vi "Forward SubVi.vi"(10 "Numeric":i32, 11 "Array":cluster{"Horizontal":i32, i32}[](array[cluster])) -> (2 "Cluster 2":cluster{"Horizontal":dbl, dbl}, 3 "Cluster":cluster{"Horizontal":i32, i32})   [LabVIEW 2014]
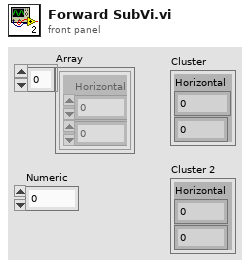
[diagram p1: front panel]
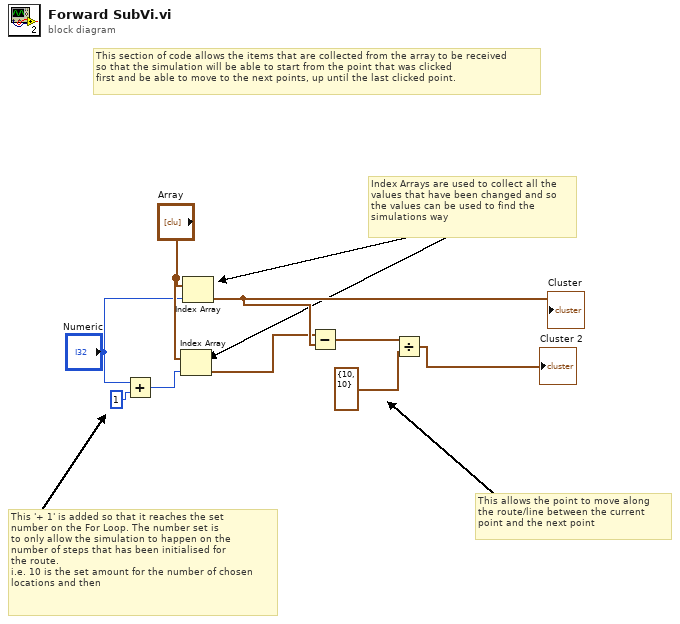
[diagram p0: block diagram]
diagram:
  # "This section of code allows the items that are collected from the array to be received\nso that the simulation will be able to start from the point that was clicked \nfirst and be able to move to the next points, up until the last clicked point."
  # "This '+ 1' is added so that it reaches the set\nnumber on the For Loop. The number set is \nto only allow the simulation to happen on the\nnumber of steps that has been initialised for \nthe route. \ni.e. 10 is the set amount for the number of chosen \nlocations and then"
  # "This allows the point to move along \nthe route/line between the current\npoint and the next point"
  # "Index Arrays are used to collect all the\nvalues that have been changed and so \nthe values can be used to find the \nsimulations way"
  n1 = Add(x="Numeric", y=1) -> (x+y=w3:i32)
  n2 = Index Array(array="Array", index=w3) -> (element=w7:cluster{"Horizontal":i32, i32})
  n3 = Index Array(array="Array", index="Numeric") -> (element=w8:cluster{"Horizontal":i32, i32})
  "Cluster" <- w8
  n4 = Subtract(x=w7, y=w8) -> (x-y=w4:cluster{"Horizontal":i32, i32})
  n5 = Divide(x=w4, y=cluster{"Horizontal":i32, i32} {"Horizontal"=10, 10}) -> (x/y=→"Cluster 2":cluster{"Horizontal":dbl, dbl})
